vi "Configure Connection.vi"(8 "error in":errorcluster, 11 "Acopian in":refnum<class "Acopian.lvclass">) -> (0 "error out":errorcluster, 3 "Acopian out":refnum<class "Acopian.lvclass">)   [LabVIEW 2019, in "Acopian.lvlib" / "Acopian.lvclass"]
uses:
  Library/Acopian.lvclass
  Library/Acopian.lvclass/Acopian.ctl
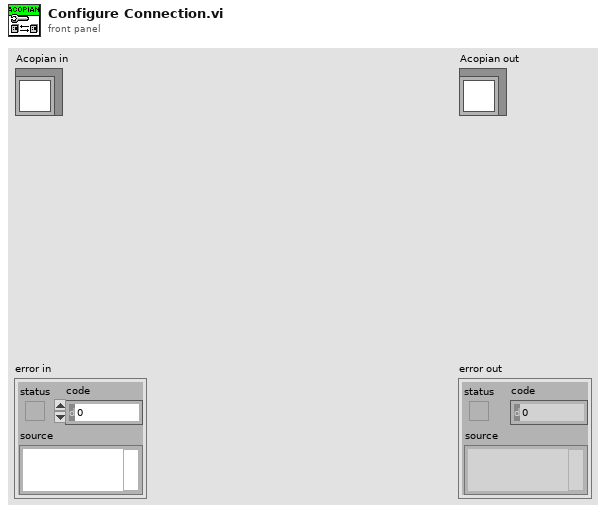
[diagram p1: front panel]
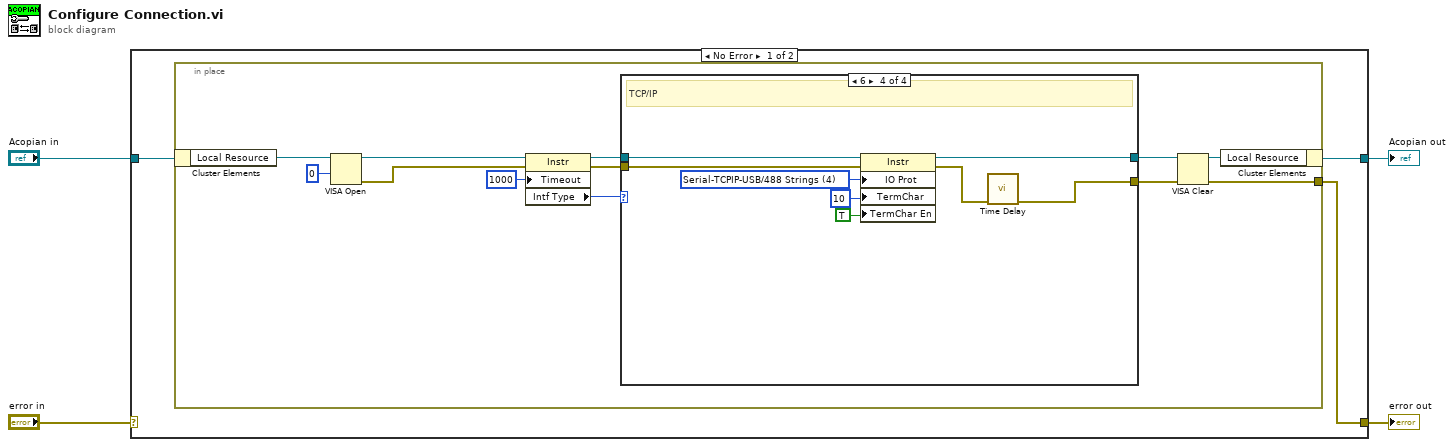
[diagram p0: block diagram]
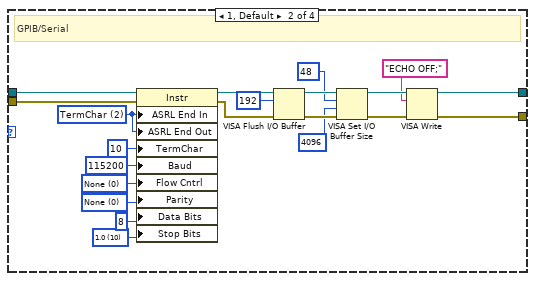
[diagram p3: hidden frame]
diagram:
  n1 = case shown="No Error" "error in" {
    selector: "error in" -> [_ w54]
    tunnel: [w5 w54] -> w3
    tunnel: [w6 w53] -> w1
    tunnel: "Acopian in" -> [w7 w53]
    frame No Error {
      n2 = in-place {
        in-place-border: [w8] -> w5
        n3 = in-place-cluster #1(w7) -> ("Local Resource"=w13:refnum<visa-resource-name>)
        n4 = VISA Open(access mode=u32 0, VISA resource name=w13) -> (VISA resource name=w12:refnum<visa-resource-name>, error out=w11:errorcluster)  [unwired: 3 in]
        n5 = property class="Instr"(reference=w12, error in=w11, "Timeout"=u32 1000 ("General Settings:Timeout Value")) -> (reference out=w18:refnum<visa-resource-name>, error out=w15:errorcluster, "Intf Type"=w19:u16)
        n6 = case shown="6" w19 {
          tunnel: w18 -> [w21 w42 w44 w52]
          tunnel: [w21 w22 w44 w47] -> w16
          tunnel: w15 -> [w20 w41 w43 w51]
          tunnel: [w20 w23 w43 w45] -> w9
          frame 0 {
            # "unrecognized Values"
          }
          frame 1, Default {
            w34 = u16 10 items=["1.0"=10, "1.5"=15, "2.0"=20] ("Serial Settings:Stop Bits")
            w36 = u16 0 items=["None", "Odd", "Even", "Mark", "Space"] ("Serial Settings:Parity")
            w37 = u16 0 items=["None", "XON/XOFF", "RTS/CTS", "XON/XOFF & RTS/CTS", "DTR/DSR", "XON/XOFF & DTR/DSR"] ("Serial Settings:Flow Control")
            w40 = u16 2 items=["None", "Last Bit", "TermChar"] ("Serial Settings:End Mode for Reads")
            # "GPIB/Serial"
            n7 = property class="Instr"(reference=w42, error in=w41, "ASRL End In"=w40, "ASRL End Out"=w40, "TermChar"=u8 10 ("Message Based Settings:Termination Character"), "Baud"=u32 115200 ("Serial Settings:Baud Rate"), "Flow Cntrl"=w37, "Parity"=w36, "Data Bits"=u16 8 ("Serial Settings:Data Bits"), "Stop Bits"=w34) -> (reference out=w25:refnum<visa-resource-name>, error out=w24:errorcluster)
            n8 = VISA Flush I/O Buffer(VISA resource name=w25, mask (16)=u16 192, error in (no error)=w24) -> (VISA resource name out=w33:refnum<visa-resource-name>, error out=w32:errorcluster)
            n9 = VISA Set I/O Buffer Size(VISA resource name=w33, mask (16)=u16 48, size (4096)=u32 4096 ("size (0)"), error in (no error)=w32) -> (VISA resource name out=w30:refnum<visa-resource-name>, error out=w31:errorcluster)
            n10 = VISA Write(VISA resource name=w30, write buffer="ECHO OFF;" ("ID Query"), error in (no error)=w31) -> (VISA resource name out=w22:refnum<visa-resource-name>, error out=w23:errorcluster)  [unwired: 1 out]
          }
          frame 2 {
            # "GPIB-VXI"
          }
          frame 6 {
            w50 = u16 4 items=["Normal"=1, "VXI/FDC"=2, "GPIB/HS488"=3, "Serial-TCPIP-USB/488 Strings"=4, "USBTMC/Vendor-Specific"=5] ("Message Based Settings:IO Protocol")
            # "TCP/IP"
            n11 = property class="Instr"(reference=w52, error in=w51, "IO Prot"=w50, "TermChar"=u8 10 ("Message Based Settings:Termination Character"), "TermChar En"=TRUE ("Message Based Settings:Termination Character Enable")) -> (reference out=w47:refnum<visa-resource-name>, error out=w46:errorcluster)
            n12 = call "Time Delay"("error in (no error)"=w46) -> ("error out"=w45:errorcluster)  [unwired: 10 in]
          }
        }
        n13 = VISA Clear(VISA resource name=w16, error in (no error)=w9) -> (VISA resource name out=w10:refnum<visa-resource-name>, error out=w8:errorcluster)
        n14 = in-place-cluster #1("Local Resource"=w10) -> (w6:refnum<class "Acopian.lvclass">)
      }
    }
    frame Error {
    }
  }
  "error out" <- w3
  "Acopian out" <- w1
